vi "Load Saved Devices.vi"(8 "error in":errorcluster) -> (0 "error out":errorcluster, 4 "Menu Devices":string[](array[string]))   [LabVIEW 2024, in "Data Base.lvlib"]
uses:
  Data Base.lvlib
  <vilib>/Utility/config.llb/Read Key (String).vi
  Support/General Type Defs/Global Data.vi
  <vilib>/Utility/config.llb/NI_LVConfig.lvlib
  Support/General Type Defs/General Type Defs.lvlib
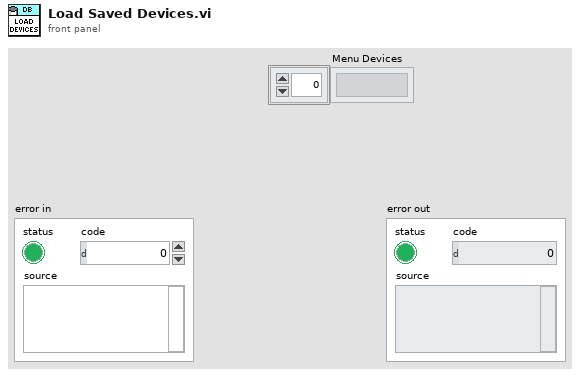
[diagram p1: front panel]
types:
  T1 = typedef "NI_LVConfig.lvlib/Config Data RefNum.ctl" = refnum<k1>
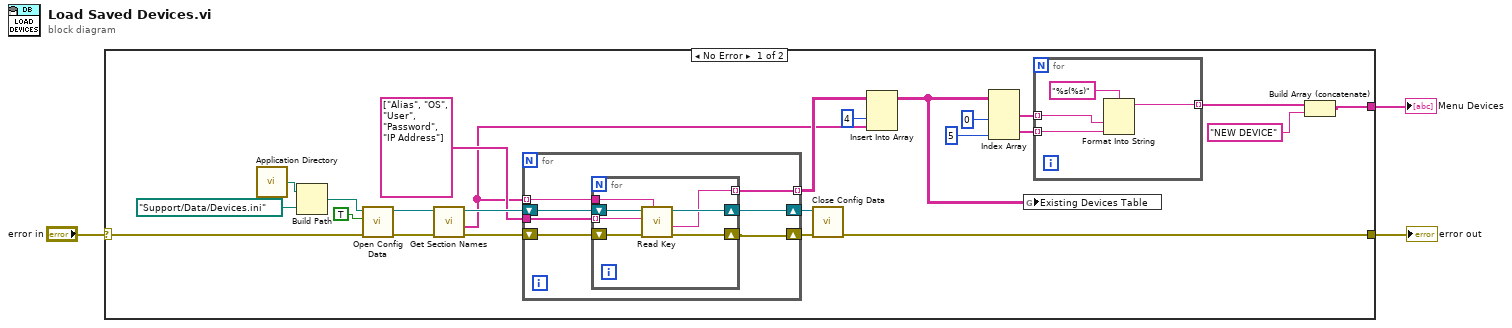
[diagram p0: block diagram]
diagram:
  n1 = case shown="No Error" "error in" {
    selector: "error in" -> [w15 w46]
    tunnel: [w16 w46] -> w3
    tunnel: [w4 _] -> w1
    frame No Error {
      n2 = call <vilib>:"Application Directory.vi"() -> ("Application Directory"=w27:path)
      n3 = Build Path(base path=w27, name or relative path=path "Support/Data/Devices.ini") -> (appended path=w25:path)
      n4 = call <vilib>:"Open Config Data.vi"("error in (no error)"=w15, "create file if necessary (T)"=TRUE, "configuration file path"=w25) -> ("error out"=w20:errorcluster, "refnum"=w23:T1)  [unwired: 6 in, 1 out]
      n5 = call <vilib>:"Get Section Names.vi"("error in (no error)"=w20, "refnum"=w23) -> ("error out"=w21:errorcluster, "section names"=w12:string[], "refnum out"=w22:T1)  [unwired: 7 in]
      n6 = for {
        tunnel: w12 -> [w36] mode=indexing
        tunnel: string[] ["Alias", "OS", "User", "Password", "IP Address"] -> [w35]
        shift-right: [w33] -> w17
        shift-left: w22 -> [w38]
        shift-right: [w34] -> w18
        shift-left: w21 -> [w37]
        tunnel: [w32] -> w14 mode=indexing
        n7 = for {
          tunnel: w36 -> [w43]
          tunnel: w35 -> [w42] mode=indexing
          shift-right: [w40] -> w33
          shift-left: w38 -> [w45]
          shift-right: [w41] -> w34
          shift-left: w37 -> [w44]
          tunnel: [w39] -> w32 mode=indexing
          n8 = call-poly <vilib>:"Read Key.vi"("section"=w43, "error in (no error)"=w44, "key"=w42, "refnum"=w45) -> ("error out"=w41:errorcluster, "value"=w39:string, "refnum out"=w40:T1)  [unwired: 4 in, 1 out]
        }
      }
      n9 = call <vilib>:"Close Config Data.vi"("error in (no error)"=w18, "refnum"=w17) -> ("error out"=w16:errorcluster)  [unwired: 8 in, 1 out]
      n10 = Insert Into Array(array=w14, index (col)=4, new element=w12) -> (w5:string[][])  [unwired: 1 in]
      n11 = Index Array(array=w5, index (col) #1=0 ("index (col)"), index (col) #2=5 ("index (col)")) -> (element #1=w8:string[], element #2=w9:string[])  [unwired: 2 in]
      n12 = global write "Global Data.vi" "Existing Devices Table"(w5) -> ()
      n13 = for {
        tunnel: w8 -> [w30] mode=indexing
        tunnel: w9 -> [w29] mode=indexing
        tunnel: [w28] -> w10 mode=indexing
        n14 = Format Into String(format string="%s(%s)", w30, w29) -> (resulting string=w28:string)  [unwired: 2 in, 1 out]
      }
      n15 = Build Array (concatenate)(w10, "NEW DEVICE" ("format string")) -> (w4:string[])
    }
    frame Error {
    }
  }
  "error out" <- w3
  "Menu Devices" <- w1
